vi "mso7014b_init_self_test.vi"() -> (1 "error out":errorcluster, 2 "VISA resource name out":refnum<visa-resource-name>)   [LabVIEW 2016]
uses:
  <instrlib>/Agilent 6000 Series/Public/Configure/Configure Edge Trigger Source.vi
  <instrlib>/Agilent 6000 Series/Public/Data/Read Single Waveform.vi
  <instrlib>/Agilent 6000 Series/Agilent 6000 Series.lvlib
panel:
  out "簇数组":cluster{"Waveform Data":waveform(dbl)}[](array[cluster])
  out "Waveform":waveform(dbl)
  out "Waveform Data":waveform(dbl)(graph)
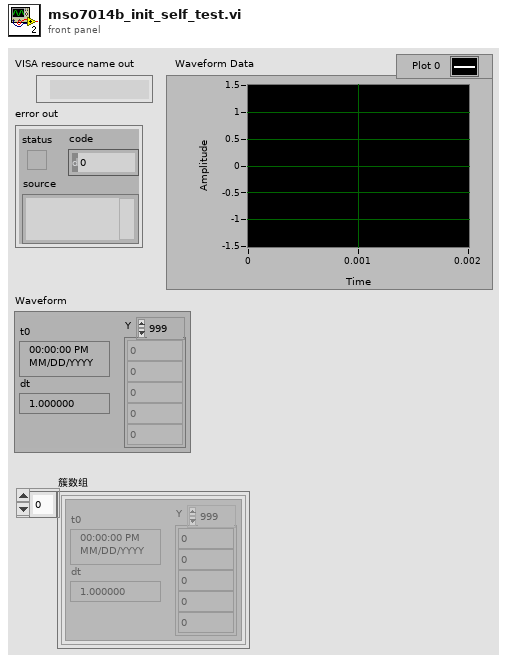
[diagram p1: front panel]
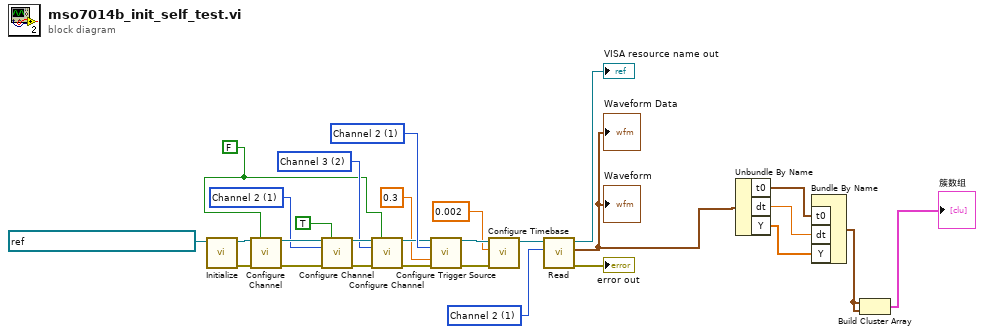
[diagram p0: block diagram]
diagram:
  w9 = u16 1 items=["Channel 1", "Channel 2", "Channel 3", "Channel 4", "Math"] ("Source (0: Channel 1)")
  w19 = u16 1 items=["Channel 1", "Channel 2", "Channel 3", "Channel 4", "DIG 0", "DIG 1", "DIG 2", "DIG 3", "DIG 4", "DIG 5", "DIG 6", "DIG 7", "DIG 8", "DIG 9", "DIG 10", "DIG 11", "DIG 12", "DIG 13", "DIG 14", "DIG 15", "Line", "External"] ("Trigger Source (0: Channel 1)")
  w20 = FALSE ("Enable Channel (T: Enable)")
  w23 = u16 2 items=["Channel 1", "Channel 2", "Channel 3", "Channel 4"] ("Channel (0: Channel 1)")
  w25 = u16 1 items=["Channel 1", "Channel 2", "Channel 3", "Channel 4"] ("Channel (0: Channel 1)")
  n1 = call <instrlib>:"Initialize.vi"("VISA resource name"=refnum<visa-resource-name> "tcpip0::192.168.40.220::instr") -> ("error out"=w17:errorcluster, "VISA resource name out"=w18:refnum<visa-resource-name>)  [unwired: 9 in]
  n2 = call <instrlib>:"Configure Channel.vi"("VISA resource name"=w18, "Enable Channel (T: Enable)"=w20, "error in (no error)"=w17) -> ("VISA resource name out"=w27:refnum<visa-resource-name>, "error out"=w22:errorcluster)  [unwired: 11 in]
  n3 = call <instrlib>:"Configure Channel.vi"("VISA resource name"=w27, "Enable Channel (T: Enable)"=TRUE, "Channel (0: Channel 1)"=w25, "error in (no error)"=w22) -> ("VISA resource name out"=w26:refnum<visa-resource-name>, "error out"=w21:errorcluster)  [unwired: 10 in]
  n4 = call <instrlib>:"Configure Channel.vi"("VISA resource name"=w26, "Enable Channel (T: Enable)"=w20, "Channel (0: Channel 1)"=w23, "error in (no error)"=w21) -> ("VISA resource name out"=w16:refnum<visa-resource-name>, "error out"=w15:errorcluster)  [unwired: 10 in]
  n5 = call-poly <instrlib>:"Configure Trigger Source.vi"("VISA resource name"=w16, "Trigger Source (0: Channel 1)"=w19, "Trigger Level (0.0 V)"=0.3, "error in (no error)"=w15) -> ("VISA resource name out"=w14:refnum<visa-resource-name>, "error out"=w13:errorcluster)  [unwired: 10 in]
  n6 = call <instrlib>:"Configure Timebase.vi"("error in (no error)"=w13, "Timebase (20.0E-9)"=0.002, "VISA resource name"=w14) -> ("VISA resource name out"=w10:refnum<visa-resource-name>)  [unwired: 7 in, 1 out]
  n7 = call-poly <instrlib>:"Read.vi"("Source (0: Channel 1)"=w9, "VISA resource name"=w10) -> ("error out"=→"error out":errorcluster, "Waveform Data"=w1:waveform(dbl), "VISA resource name out"=→"VISA resource name out":refnum<visa-resource-name>)  [unwired: 7 in]
  "Waveform Data" <- w1
  "Waveform" <- w1
  n8 = Unbundle By Name(w1) -> ("t0"=w6:timestamp, "dt"=w5:dbl, "Y"=w4:dbl[])
  n9 = Bundle By Name("t0"=w6, "dt"=w5, "Y"=w4) -> (w3:waveform(dbl))  [unwired: 1 in]
  n10 = Build Cluster Array(w3, w3) -> (→"簇数组":cluster{waveform(dbl)}[])
